vi "Up_ImgToReal.vi"(10 "GrayImg":string, 11 "Array":cluster{"R_X":dbl, "R_Y":dbl}[](array[cluster])) -> (1 "pos2":cluster{"X":sgl, "Y":sgl}, 2 "angle":sgl, 3 "pos1":cluster{"X":sgl, "Y":sgl})   [LabVIEW 2019]
uses:
  <vilib>/vision/NI_Vision_Development_Module.lvlib
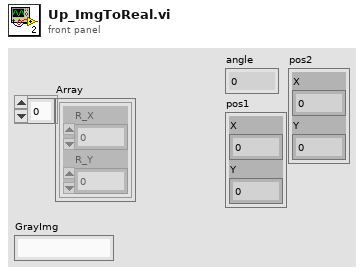
[diagram p1: front panel]
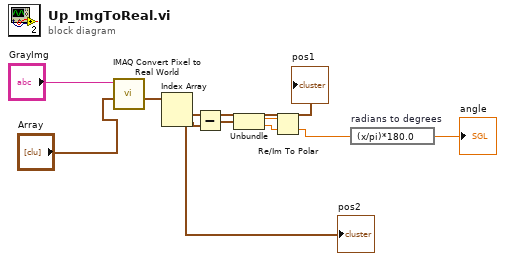
[diagram p0: block diagram]
diagram:
  n1 = call "IMAQ Convert Pixel to Real World"("Array of Pixel Coordinates"="Array", "Calibrated Image"="GrayImg") -> ("Array of Real World Coordinates"=w7:cluster{"X":sgl, "Y":sgl}[])  [unwired: 4 in, 5 out]
  n2 = Index Array(array=w7) -> (element #1=w2:cluster{"X":sgl, "Y":sgl}, element #2=w1:cluster{"X":sgl, "Y":sgl})  [unwired: 2 in]
  "pos1" <- w2
  "pos2" <- w1
  n3 = Subtract(x=w2, y=w1) -> (x-y=w8:cluster{"X":sgl, "Y":sgl})
  n4 = Unbundle(w8) -> ("X"=w9:sgl, "Y"=w10:sgl)
  n5 = Re/Im To Polar(2:w10, 3:w9) -> (0:w4:sgl)  [unwired: 1 out]
  n6 = expression code="(x/pi)*180.0" "radians to degrees"(w4) -> (→"angle":sgl)
